vi "Auto Setup.vi"() -> ()   [LabVIEW 2019]
uses:
  Types/Path Data.ctl
  <vilib>/Rock Robotics/WPI/DriverStation/WPI_DriverStationRobotMode2.ctl
  27e1c827-0946-466c-bb8f-e5127fca4b7b.vi
  22df871f-6e36-4dee-8847-80ba77881a4a.vi
  Framework/Robot Global Data.vi
  <vilib>/Rock Robotics/Network Tables/NT Write String Array.vi
panel:
  out "error out":errorcluster
  in  "override":bool=TRUE
  in  "error in":errorcluster
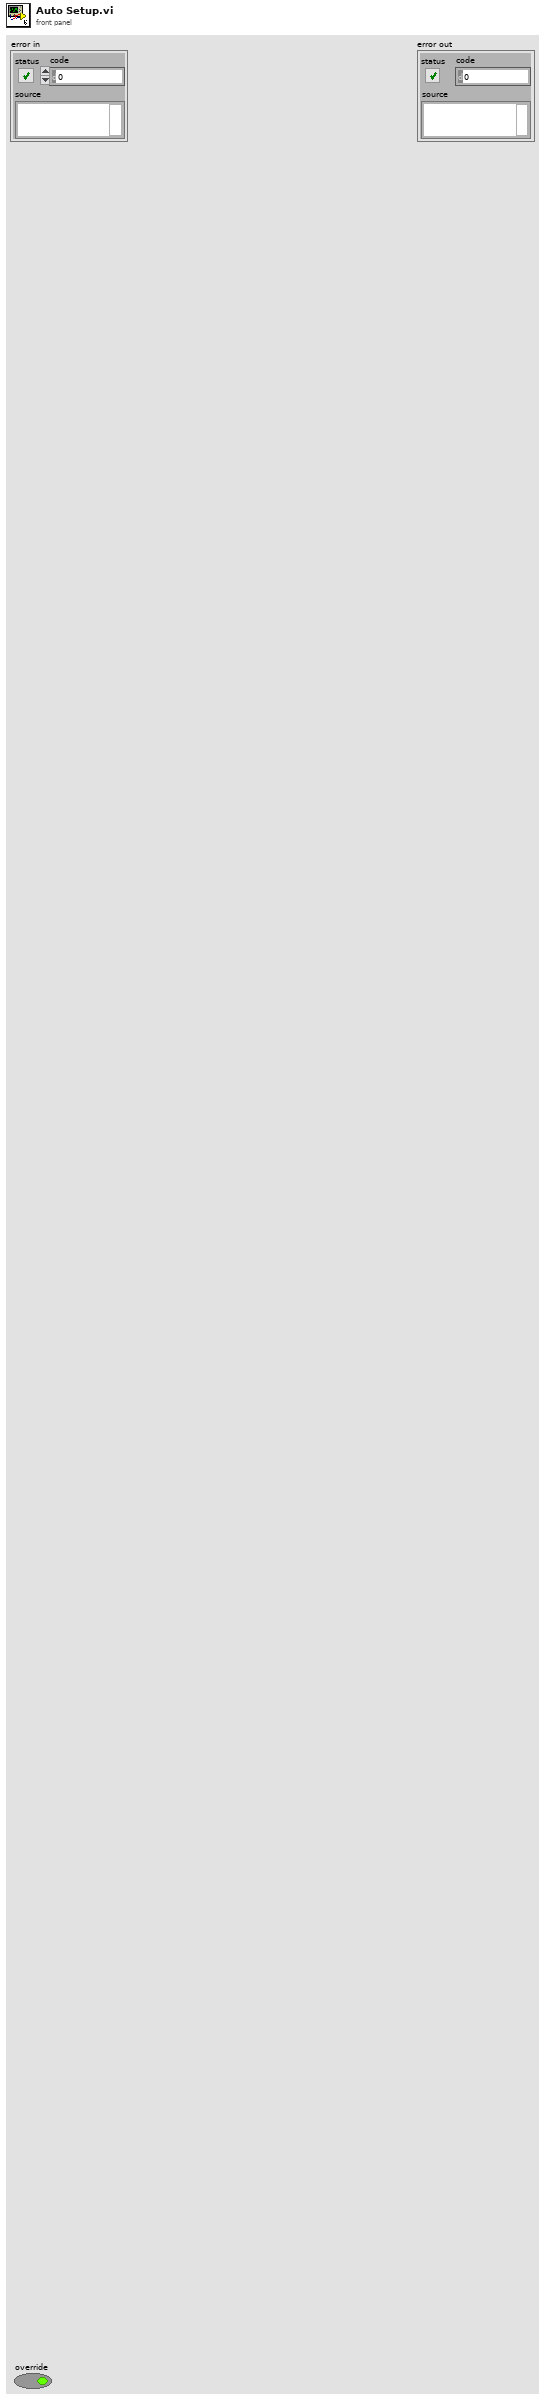
[diagram p1: front panel]
types:
  T1 = typedef "Path Data.ctl" = cluster{"Trajectory Data":cluster{"Segment Name":string, "Type":enum16{"Accel Straight", "Const Straight", "Blend", "Circle"}, "Traj Pos Points":cluster{"x":dbl, "y":dbl, "th":dbl}[], "Traj Vel Points":cluster{"V":dbl, "th":dbl}[], "Accel Index":i32, "Decel Index":i32}[]}[]
  T2 = typedef "WPI_DriverStationRobotMode2.ctl" = enum16{"Autonomous Disabled", "Autonomous Enabled", "Teleop Disabled", "Teleop Enabled", "Disconnected", "Finish", "Test Disabled", "Test Enabled", "Emergency Stopped"}
  T3 = cluster{"Segment Name":string, "Type":enum16{"Accel Straight", "Const Straight", "Blend", "Circle"}, "Traj Pos Points":cluster{"x":dbl, "y":dbl, "th":dbl}[], "Traj Vel Points":cluster{"V":dbl, "th":dbl}[], "Accel Index":i32, "Decel Index":i32}[]
  T4 = cluster{"Trajectory Data":cluster{"Segment Name":string, "Type":enum16{"Accel Straight", "Const Straight", "Blend", "Circle"}, "Traj Pos Points":cluster{"x":dbl, "y":dbl, "th":dbl}[], "Traj Vel Points":cluster{"V":dbl, "th":dbl}[], "Accel Index":i32, "Decel Index":i32}[]}
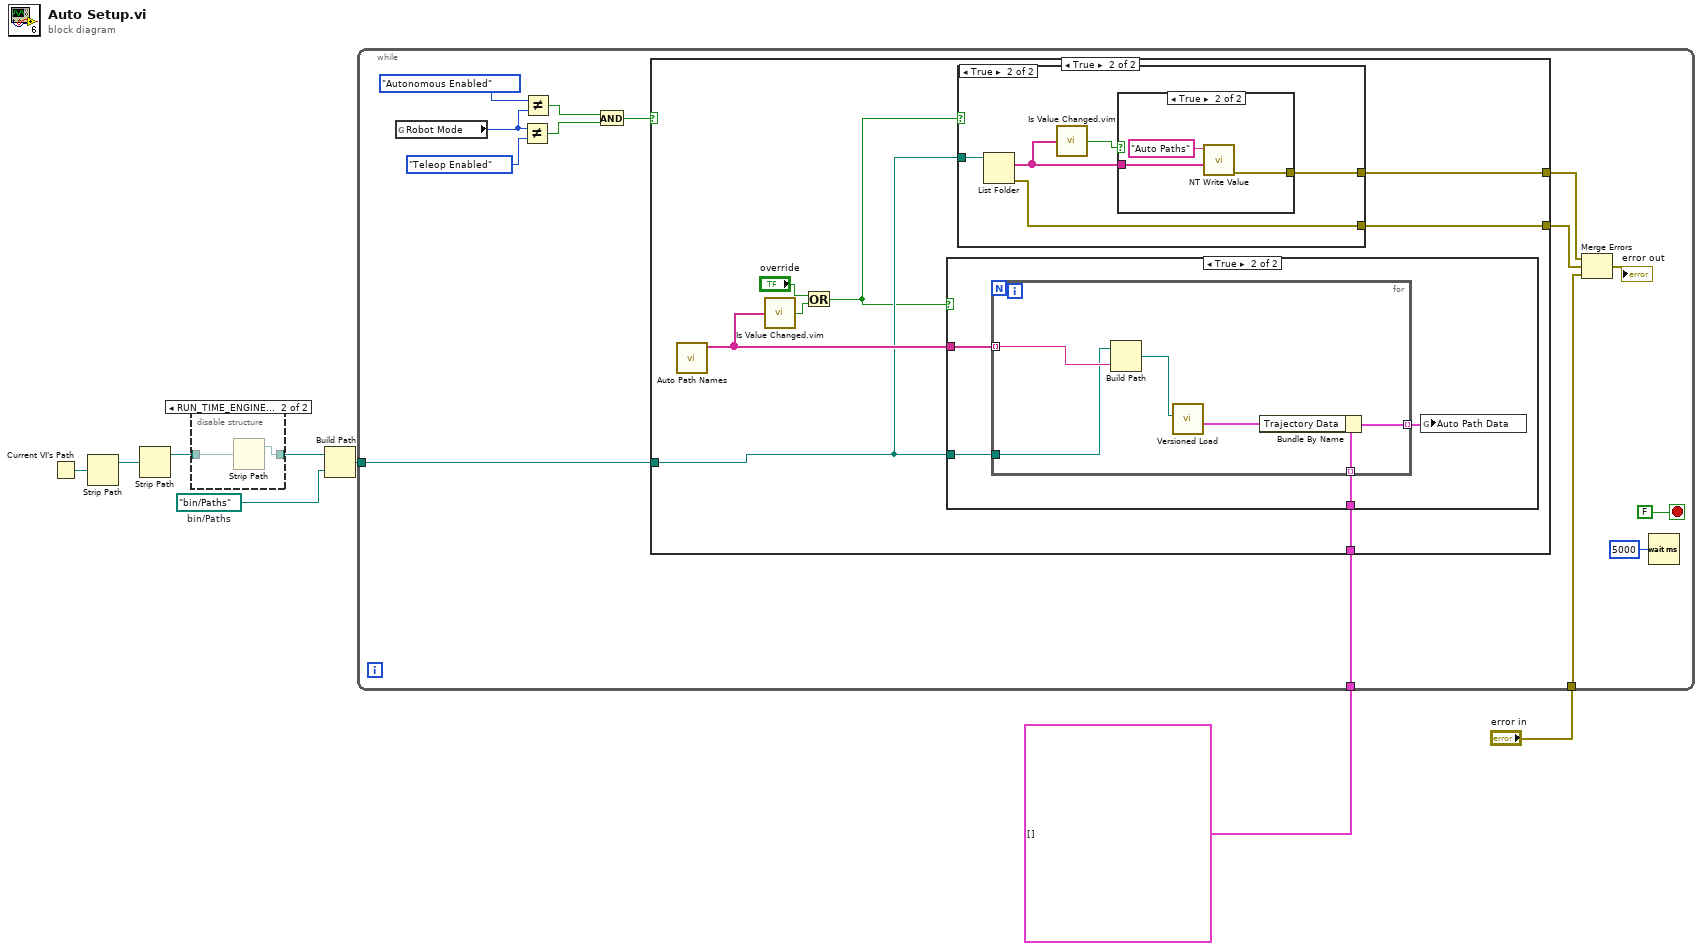
[diagram p0: block diagram]
diagram:
  w3 = path "bin/Paths"  # bin/Paths
  n1 = Current VI's Path() -> (path=w4:path)
  n2 = Strip Path(path=w4) -> (stripped path=w5:path)  [unwired: 1 out]
  n3 = Strip Path(path=w5) -> (stripped path=w7:path)  [unwired: 1 out]
  n4 = disable-structure shown="RUN_TIME_ENGINE==True, Default" {
    disable-tunnel: [w9 w10] -> w6
    disable-tunnel: w7 -> [w9 w11]
    frame condition #0 (active) {
    }
    frame condition #1 {
      n5 = Strip Path(path=w11) -> (stripped path=w10:path)  [unwired: 1 out]
    }
  }
  n6 = Build Path(base path=w6, name or relative path=w3) -> (appended path=w2:path)
  n7 = while {
    tunnel: "error in" -> [w13]
    tunnel: w2 -> [w17]
    tunnel: T1 [] ("Array") -> [w14]
    stop <- FALSE stop-if-true
    n8 = global read "Robot Global Data.vi" "Robot Mode"() -> (w23:T2)
    n9 = Not Equal?(x=w23, y=WPI_DriverStationRobotMode2."Teleop Enabled") -> (x != y?=w20:bool)
    n10 = Not Equal?(x=WPI_DriverStationRobotMode2."Autonomous Enabled", y=w23) -> (x != y?=w21:bool)
    n11 = And(x=w21, y=w20) -> (x .and. y?=w12:bool)
    n12 = case shown="True" w12 {
      tunnel: w17 -> [_ w30]
      tunnel: [_ w29] -> w16
      tunnel: [_ w28] -> w15
      tunnel: w14 -> [_ w27]
      frame False {
      }
      frame True {
        n13 = call "Auto Path Names.vi"() -> ("Path Names"=w31:string[])  [unwired: 11 in]
        n14 = call "Is Value Changed.vim"("value"=w31) -> ("changed or first call?"=w33:bool)
        n15 = Or(x="override", y=w33) -> (x .or. y?=w26:bool)
        n16 = case shown="True" w26 {
          tunnel: w31 -> [_ w45]
          tunnel: w30 -> [_ w44]
          tunnel: w27 -> [_ w43]
          frame False {
          }
          frame True {
            n17 = for {
              tunnel: w45 -> [w51] mode=indexing
              tunnel: w44 -> [w49]
              tunnel: w43 -> [w48] mode=indexing
              tunnel: [w46] -> w42 mode=indexing
              n18 = Build Path(base path=w49, name or relative path=w51) -> (appended path=w50:path)
              n19 = call "Versioned Load.vi"("path"=w50) -> ("Trajectory Data"=w47:T3)  [unwired: 4 in, 6 out]
              n20 = Bundle By Name(cluster=w48, "Trajectory Data"=w47) -> (w46:T4)
            }
            n21 = global write "Robot Global Data.vi" "Auto Path Data"(w42) -> ()
          }
        }
        n22 = case shown="True" w26 {
          tunnel: w30 -> [_ w38]
          tunnel: [_ w35] -> w29
          tunnel: [_ w34] -> w28
          frame False {
          }
          frame True {
            n23 = List Folder(path=w38) -> (filenames=w37:string[], error out=w34:errorcluster)  [unwired: 3 in, 2 out]
            n24 = call "Is Value Changed.vim"("value"=w37) -> ("changed or first call?"=w36:bool)
            n25 = case shown="True" w36 {
              tunnel: w37 -> [_ w40]
              tunnel: [_ w39] -> w35
              frame False {
              }
              frame True {
                n26 = call-poly <vilib>:"NT Write Value.vi"("String Array"=w40, "Name"="Auto Paths") -> ("error out"=w39:errorcluster)  [unwired: 9 in]
              }
            }
          }
        }
      }
    }
    n27 = Merge Errors(w16, w15, w13) -> (→"error out":errorcluster)
    n28 = Wait (ms)(milliseconds to wait=u32 5000) -> ()  [unwired: 1 out]
  }
